vi "Simulate Rope Data.vi"(1 "Use Buggy Movement?":bool, 2 "#Knots":i32, 3 "Moves":string[](array[string])) -> (0 "Rope Data":T1)   [LabVIEW 2020, in "AoC 2022.lvlib"]
uses:
  AoC 2022.lvlib
  Rope Data.ctl
  Positions.ctl
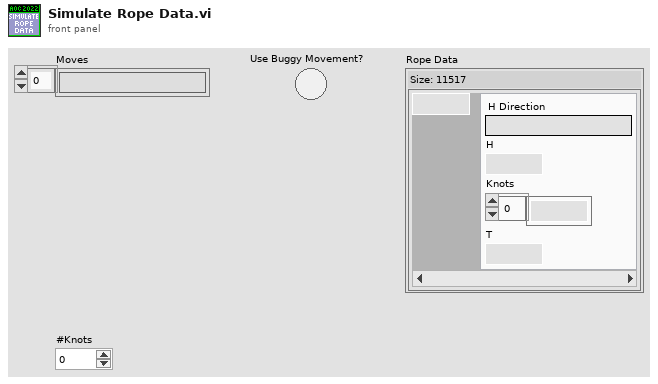
[diagram p1: front panel]
types:
  T1 = typedef "AoC 2022.lvlib/Rope Data.ctl" = map{i32, T2}
  T2 = typedef "AoC 2022.lvlib/Positions.ctl" = cluster{"H Direction":string, "H":cdb, "Knots":cdb[], "T":cdb}
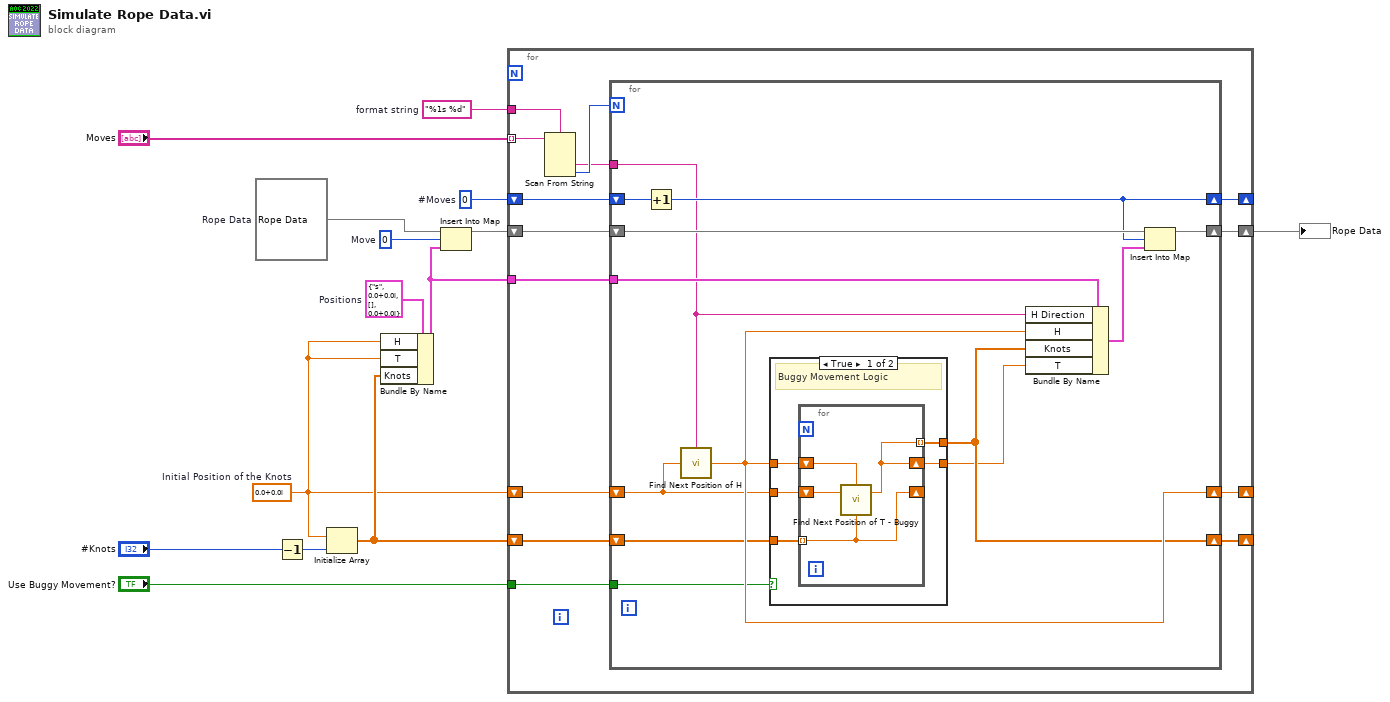
[diagram p0: block diagram]
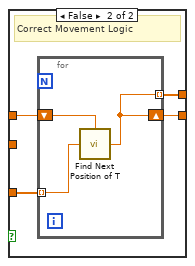
[diagram p2: hidden frame]
diagram:
  w2 = cdb 0.0+0.0i  # Initial Position of the Knots
  w5 = T1 {}  # Rope Data
  w7 = T2 {"H Direction"="s", "H"=0.0+0.0i, "Knots"=[], "T"=0.0+0.0i}  # Positions
  w4 = 0  # Move
  w10 = 0  # #Moves
  w9 = "%1s %d"  # format string
  n1 = Decrement(x="#Knots") -> (x-1=w12:i32)
  n2 = Initialize Array(w2, w12) -> (w13:cdb[])
  n3 = Bundle By Name(cluster=w7, "H"=w2, "T"=w2, "Knots"=w13) -> (w3:T2)
  n4 = Insert Into Map(map in=w5, key=w4, value=w3) -> (map out=w6:T1)  [unwired: 2 out]
  n5 = for {
    tunnel: "Moves" -> [w28] mode=indexing
    tunnel: w9 -> [w27]
    shift-right: [w24] -> _
    shift-left: w10 -> [w23]
    shift-right: [w21] -> w14
    shift-left: w6 -> [w22]
    tunnel: w3 -> [w20]
    shift-right: [w18] -> _
    shift-left: w2 -> [w19]
    shift-right: [w17] -> _
    shift-left: w13 -> [w16]
    tunnel: "Use Buggy Movement?" -> [w15]
    n6 = Scan From String(format string=w27, input string=w28) -> (output 1=w25:string, output 2=w26:i32)  [unwired: 4 in, 3 out]
    n7 = for {
      N: w26 -> [_]
      tunnel: w25 -> [w36]
      shift-right: [w38] -> w24
      shift-left: w23 -> [w39]
      shift-right: [w41] -> w21
      shift-left: w22 -> [w40]
      tunnel: w20 -> [w37]
      shift-right: [w34] -> w18
      shift-left: w19 -> [w30]
      shift-right: [w32] -> w17
      shift-left: w16 -> [w33]
      tunnel: w15 -> [w29]
      n8 = Increment(x=w39) -> (x+1=w38:i32)
      n9 = call "Find Next Position of H.vi"("Current Position of H"=w30, "Movement Direction"=w36) -> ("Next Position of H"=w34:cdb)
      n10 = case shown="True" w29 {
        tunnel: w34 -> [w46 w54]
        tunnel: w33 -> [w45 w53]
        tunnel: [w44 w52] -> w32
        tunnel: [w43 w51] -> w31
        tunnel: w30 -> [w42 _]
        frame True {
          # "Buggy Movement Logic"
          n11 = for {
            tunnel: [w49] -> w44 mode=indexing
            tunnel: w45 -> [w48] mode=indexing
            shift-right: [w49] -> w43
            shift-left: w46 -> [w50]
            shift-right: [w48] -> _
            shift-left: w42 -> [w47]
            n12 = call "Find Next Position of T - Buggy.vi"("Current Position of T"=w48, "Previous Position of H"=w47, "Current Position of H"=w50) -> ("Next Position of T"=w49:cdb)  [unwired: 2 in]
          }
        }
        frame False {
          # "Correct Movement Logic"
          n13 = for {
            tunnel: [w56] -> w52 mode=indexing
            tunnel: w53 -> [w55] mode=indexing
            shift-right: [w56] -> w51
            shift-left: w54 -> [w57]
            n14 = call "Find Next Position of T.vi"("Current Position of T"=w55, "Current Position of H"=w57) -> ("Next Position of T"=w56:cdb)
          }
        }
      }
      n15 = Bundle By Name(cluster=w37, "H Direction"=w36, "H"=w34, "Knots"=w32, "T"=w31) -> (w35:T2)
      n16 = Insert Into Map(map in=w40, key=w38, value=w35) -> (map out=w41:T1)  [unwired: 2 out]
    }
  }
  "Rope Data" <- w14
